vi "TB-Options Dialog.vi"(0 "Parameters in":T6={"Low cutoff (kHz)"=0.0, "High cutoff (kHz)"=0.0, "Duration (min)"=0.0, "dB SPL"=100.0, "Waveform"=enum."Noise", "WAVfile"=path "", "refWav"=path "", "use mic correction"=FALSE, "micCorrFile"=path "", "Pistonphone Level (dB SPL)"=0.0, "Sampling rate (Hz)"=0.0, "Buffer length (s)"=0.0, "Stream mic"=FALSE, "Fine adjust"={"Max"=0.0, "Min"=0.0}, "Mic gain"=0.0, "atten"=0.0, "Allow Slack"=FALSE, "max starts"=0, "Freq (kHz)"=8.0, "Tma (s)"=0.0, "Streamed"=[], "Drive"="", "Speaker"="", "Mic"="", "Analysis"={"Method"=enum."Default", "resol (Hz)"=0.0, "nfreq"=0, "signal"=""}, "exposeAtten"=0.0, "Digital"=""}, 2 "Parent VI":refnum<vi>) -> (4 "Parameters out":T6={"Low cutoff (kHz)"=0.0, "High cutoff (kHz)"=0.0, "Duration (min)"=0.0, "dB SPL"=100.0, "Waveform"=enum."Noise", "WAVfile"=path "", "refWav"=path "", "use mic correction"=FALSE, "micCorrFile"=path "", "Pistonphone Level (dB SPL)"=0.0, "Sampling rate (Hz)"=0.0, "Buffer length (s)"=0.0, "Stream mic"=FALSE, "Fine adjust"={"Max"=0.0, "Min"=0.0}, "Mic gain"=0.0, "atten"=0.0, "Allow Slack"=FALSE, "max starts"=0, "Freq (kHz)"=8.0, "Tma (s)"=0.0, "Streamed"=[], "Drive"="", "Speaker"="", "Mic"="", "Analysis"={"Method"=enum."Default", "resol (Hz)"=0.0, "nfreq"=0, "signal"=""}, "exposeAtten"=0.0, "Digital"=""}, 8 "Canceled?":bool)   [LabVIEW 2020]
uses:
  Typedefs/TB-Parameters.ctl
  Typedefs/TB-Analysis Parameters.ctl
  epl-vi-lib/Utility VIs/Buttons/KCheckmarkBoolean 2.ctl
  epl-vi-lib/Utility VIs/Controls/KBackground Gradient/KBackground Gradient.xctl
  epl-vi-lib/Utility VIs/Slack VIs/Slack/Slack.xctl
  epl-vi-lib/Utility VIs/Controls/KTable/KTable.xctl
  Typedefs/TB-User.ctl
  db6f5269-756f-40de-ad08-04ce0dc7adfb.vi
  epl-vi-lib/Utility VIs/File IO VIs/Read Write Anything/Read Anything.vi
panel:
  in  "Tab":T1(tab)
  in  "expose atten":dbl caption="Additional exposure attenuation (dB)"
  in  "max starts":i32 caption="Max number of starts (in case of error)"
  in  "Pistonphone Level":dbl caption="Pistonphone Level (dB SPL)"
  in  "Sampling rate (Hz)":dbl
  in  "Buffer length (s)":dbl
  in  "atten":dbl caption="Global attenuation (dB)"
  in  "Tma":dbl caption="Moving average (s)"
  in  "Signal":u16(ring)
  in  "Method":T2(ring)
  in  "resol":dbl caption="Spectrum resolution (Hz)"
  in  "nspect":i32 caption="Spectrum averages"
  in  "Digital":u16(ring) caption="Digital output" items=["None", "PXI1Slot3/port0/line0", "PXI1Slot3/port0/line1", "PXI1Slot3/port0/line2", "PXI1Slot3/port0/line3", "PXI1Slot3/port0/line4", "PXI1Slot3/port0/line5", "PXI1Slot3/port0/line6", "PXI1Slot3/port0/line7", "PXI1Slot4/port0/line0", "PXI1Slot4/port0/line1", "PXI1Slot4/port0/line2", "PXI1Slot4/port0/line3", "PXI1Slot4/port0/line4", "PXI1Slot4/port0/line5", "PXI1Slot4/port0/line6", "PXI1Slot4/port0/line7"]
  in  "Microphone":u16(ring) items=["PXI1Slot2/ai0", "PXI1Slot2/ai1", "PXI1Slot3/ai0", "PXI1Slot3/ai1", "PXI1Slot3/ai2", "PXI1Slot3/ai3", "PXI1Slot3/ai4", "PXI1Slot3/ai5", "PXI1Slot3/ai6", "PXI1Slot3/ai7", "PXI1Slot4/ai0", "PXI1Slot4/ai1", "PXI1Slot4/ai2", "PXI1Slot4/ai3", "PXI1Slot4/ai4", "PXI1Slot4/ai5", "PXI1Slot4/ai6", "PXI1Slot4/ai7"]
  in  "Speaker":u16(ring) items=["PXI1Slot2/ao0", "PXI1Slot2/ao1", "PXI1Slot3/ao0", "PXI1Slot3/ao1", "PXI1Slot4/ao0", "PXI1Slot4/ao1"]
  out "Cal mic":u16(xcontrol) caption="Additional signals"
  in  "Table":u16(xcontrol) caption="Additional signals"
  in  "Stream raw data to disk":T3
  in  "Add Button":bool
  in  "Users":i32(listbox)
  in  "Slack":cluster{"config":T4, "users":T5[]}(xcontrol)
  in  "Gradient":dbl(xcontrol)
  in  "Cancel":bool
  in  "OK":bool
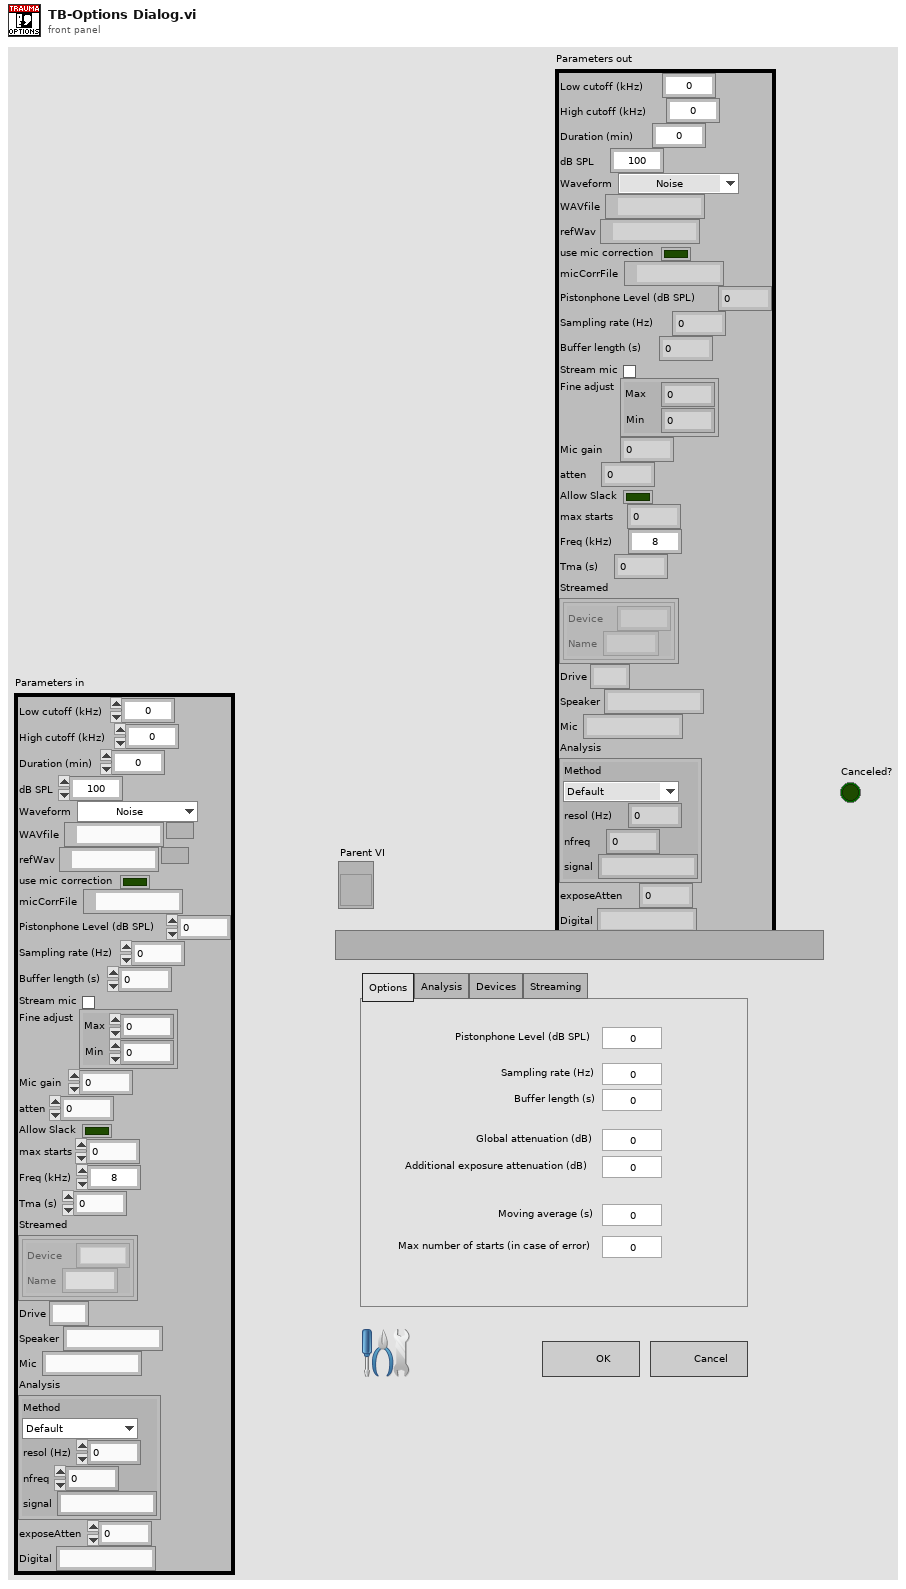
[diagram p1: front panel]
types:
  T1 = enum32{"Options", "Analysis", "Devices", "Streaming", "Slack"}
  T2 = enum16{"Default", "Periodogram", "Cross-spectrum"}
  T3 = typedef "KCheckmarkBoolean 2.ctl" = bool
  T4 = typedef "Slack-Configuration.ctl" = cluster{"app_id":string, "authed_user":cluster{"id":string}, "access_token":string, "bot_user_id":string, "team":cluster{"id":string, "name":string}, "bot channel":cluster{"id":string, "name":string}, "bot_user_name":string}
  T5 = typedef "Slack-User.ctl" = cluster{"id":string, "name":string}
  T6 = typedef "TB-Parameters.ctl" = cluster{"Low cutoff (kHz)":dbl, "High cutoff (kHz)":dbl, "Duration (min)":dbl, "dB SPL":dbl, "Waveform":enum16{"Noise", "File", "Tone"}, "WAVfile":path, "refWav":path, "use mic correction":bool, "micCorrFile":path, "Pistonphone Level (dB SPL)":dbl, "Sampling rate (Hz)":dbl, "Buffer length (s)":dbl, "Stream mic":bool, "Fine adjust":cluster{"Max":dbl, "Min":dbl}, "Mic gain":dbl, "atten":dbl, "Allow Slack":bool, "max starts":i32, "Freq (kHz)":dbl, "Tma (s)":dbl, "Streamed":cluster{"Device":string, "Name":string}[], "Drive":string, "Speaker":string, "Mic":string, "Analysis":T7, "exposeAtten":dbl, "Digital":string}
  T7 = typedef "TB-Analysis Parameters.ctl" = cluster{"Method":enum16{"Default", "Periodogram", "Cross-spectrum"}, "resol (Hz)":dbl, "nfreq":i32, "signal":string}
  T8 = enum8{"Enabled", "Disabled", "Disabled and Grayed Out"}
  T9 = typedef "TB-User.ctl" = cluster{"name":string, "id":string, "notify on errors":bool}
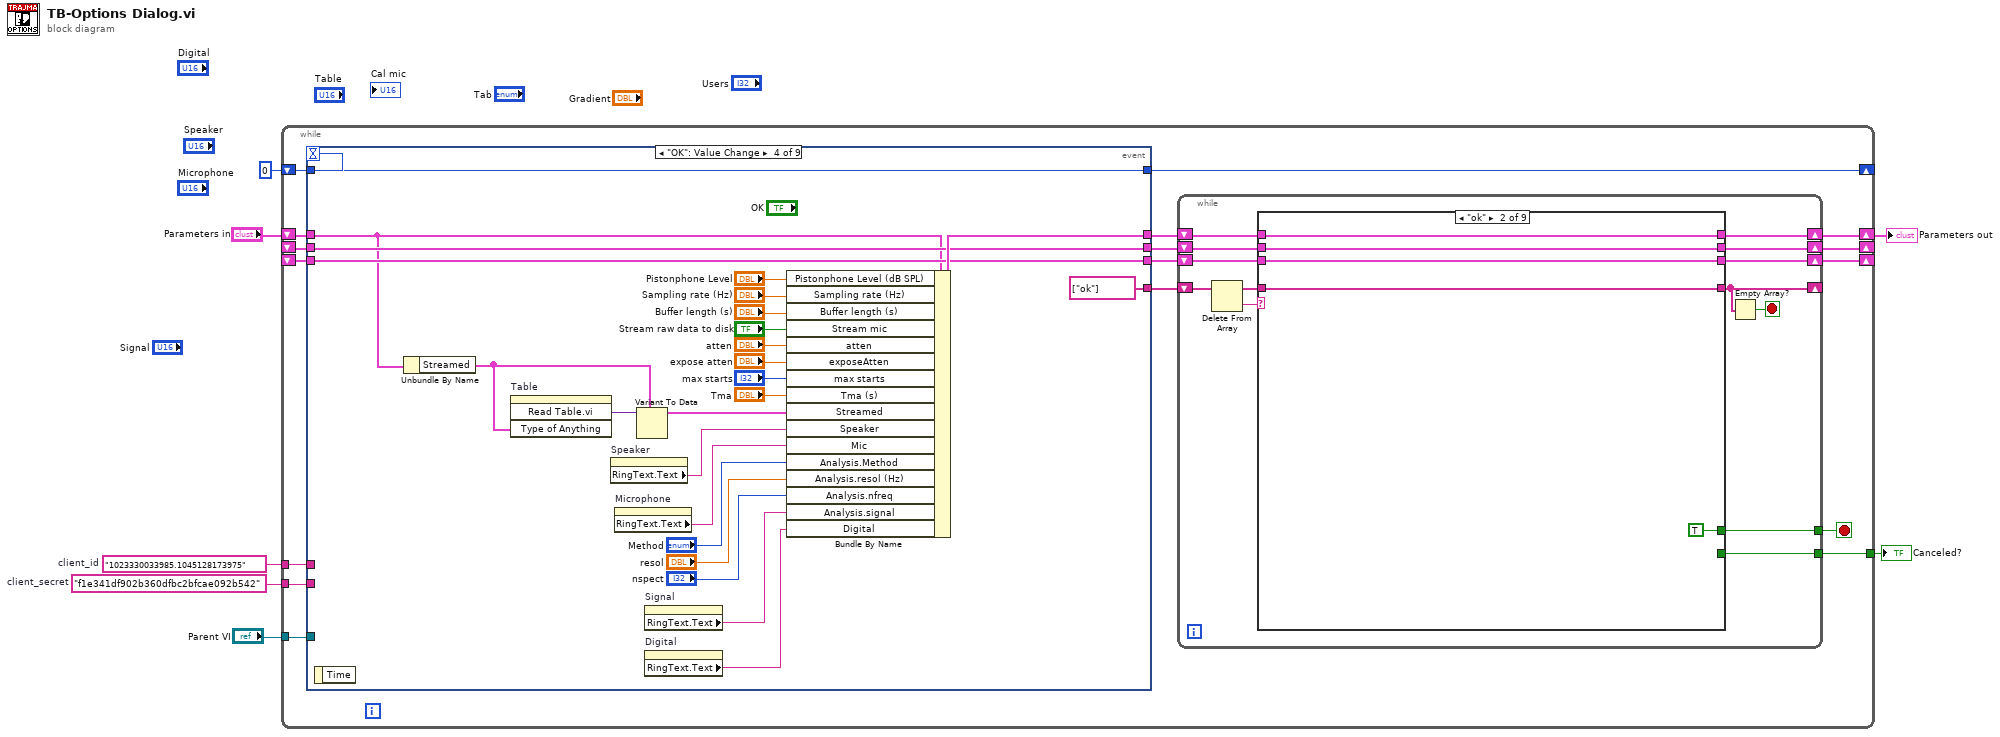
[diagram p0: block diagram]
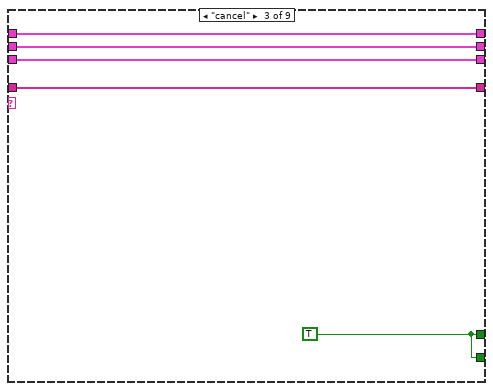
[diagram p3: hidden frame]
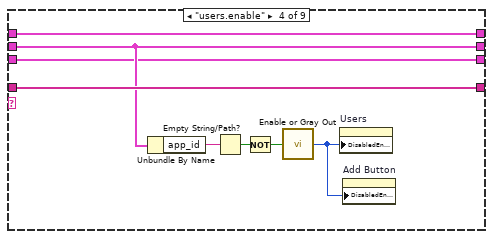
[diagram p4: hidden frame]
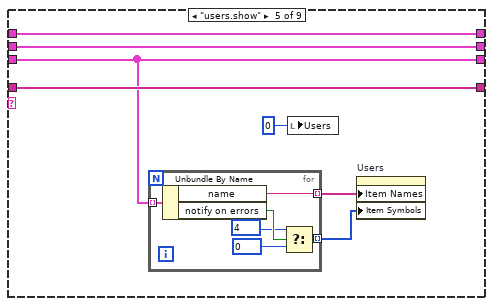
[diagram p5: hidden frame]
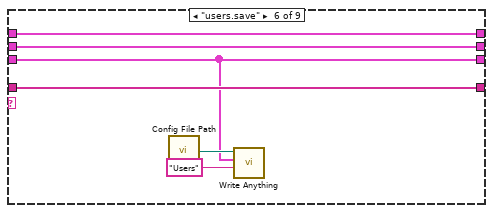
[diagram p6: hidden frame]
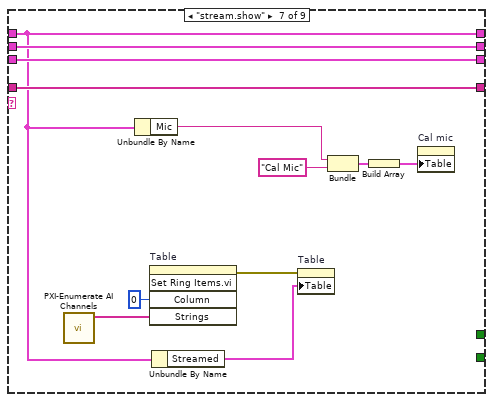
[diagram p7: hidden frame]
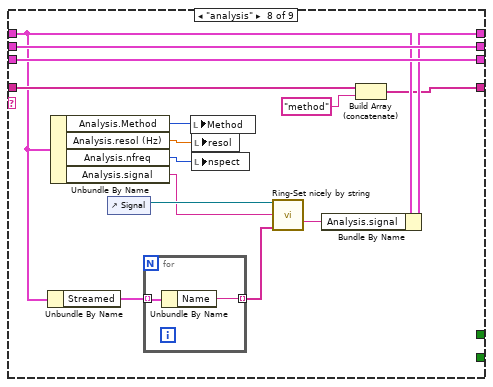
[diagram p8: hidden frame]
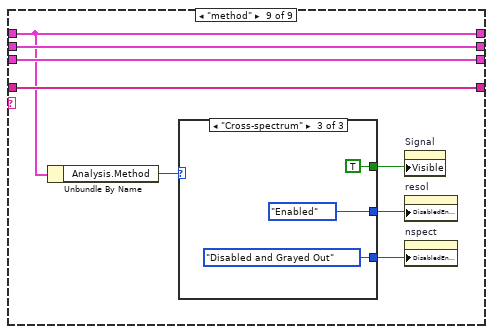
[diagram p9: hidden frame]
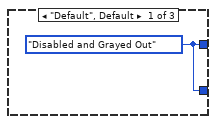
[diagram p10: hidden frame]
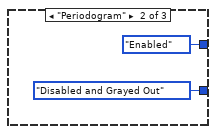
[diagram p11: hidden frame]
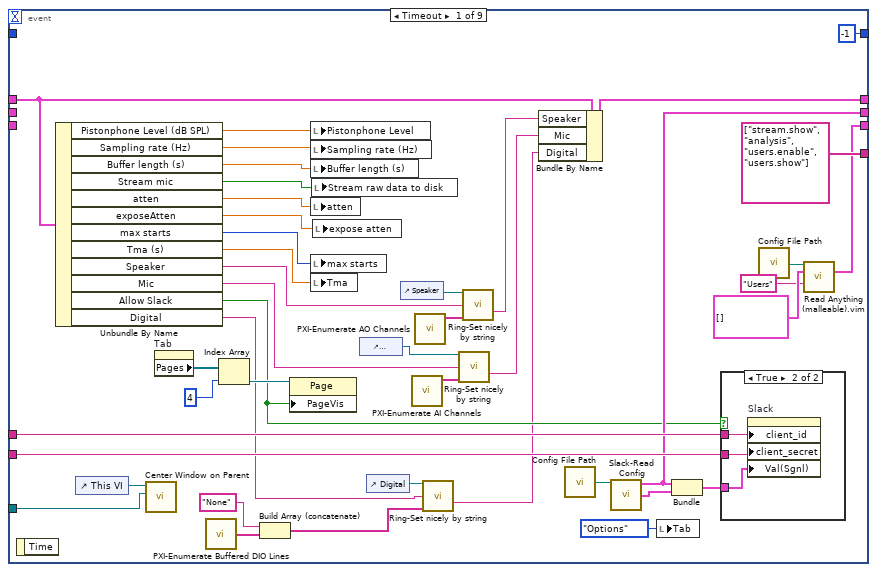
[diagram p12: hidden frame]
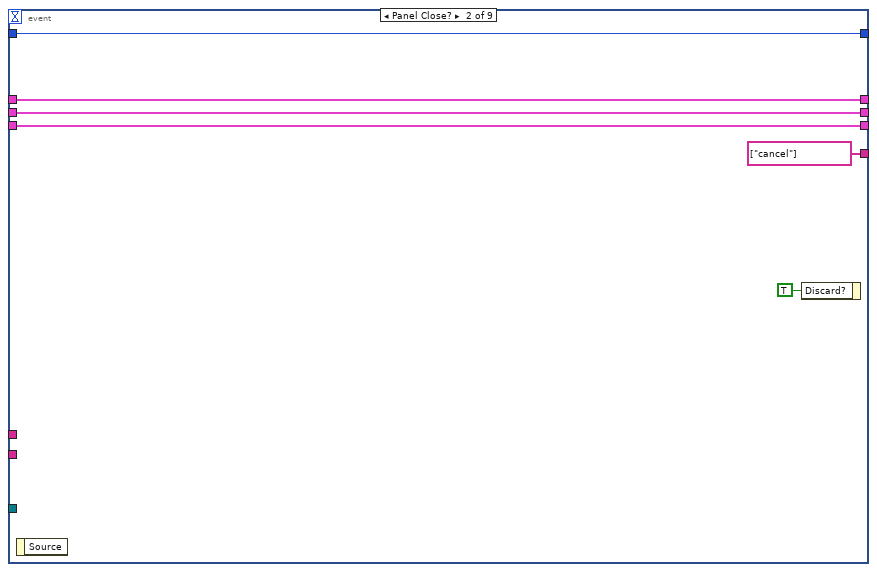
[diagram p14: hidden frame]
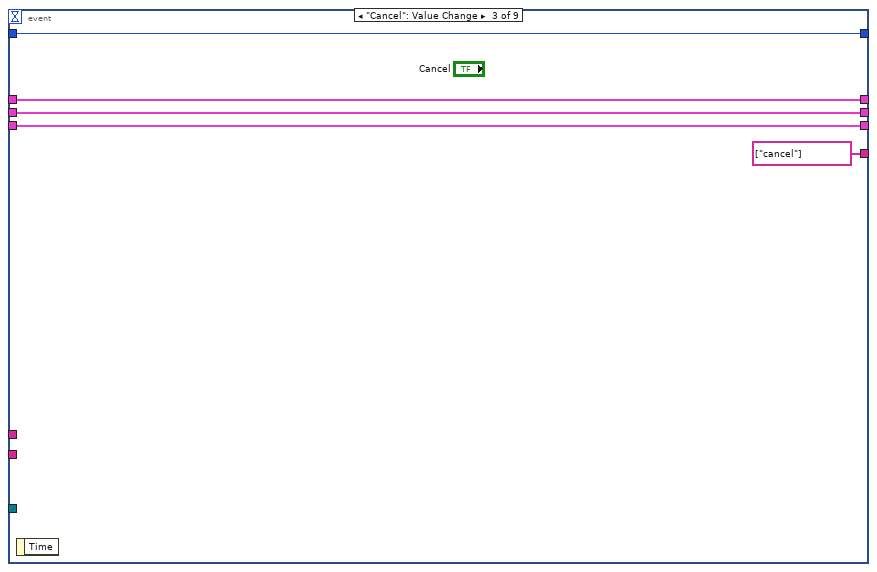
[diagram p15: hidden frame]
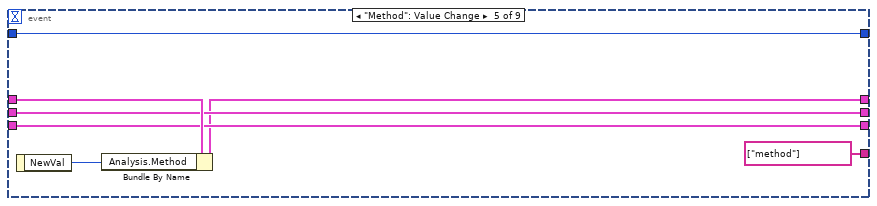
[diagram p16: hidden frame]
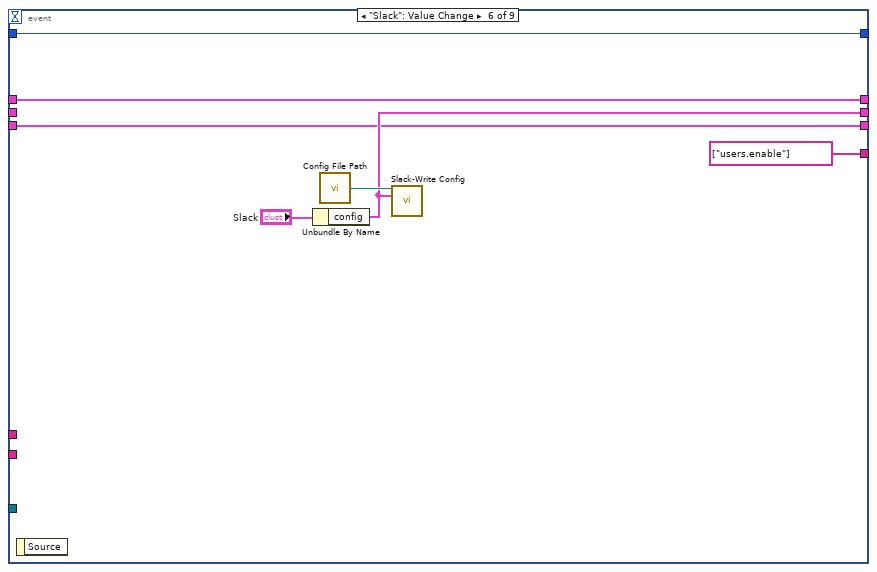
[diagram p17: hidden frame]
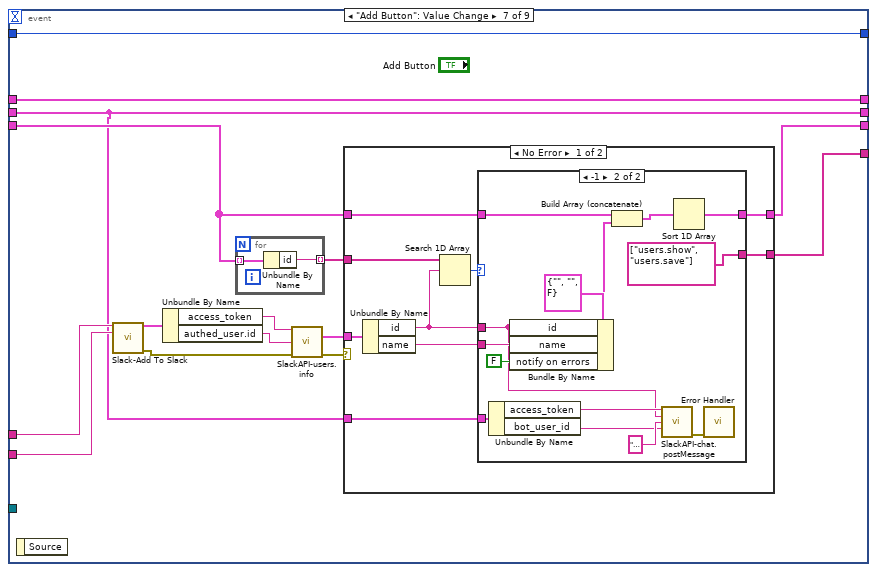
[diagram p18: hidden frame]
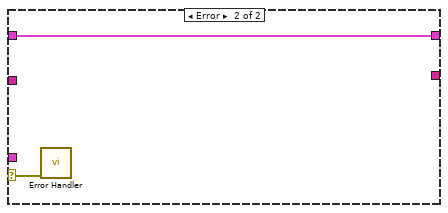
[diagram p20: hidden frame]
diagram:
  w1 = "f1e341df902b360dfbc2bfcae092b542"  # client_secret
  w2 = "1023330033985.1045128173975"  # client_id
  n1 = while {
    shift-right: [w24] -> _
    shift-left: 0 -> [w21]
    tunnel: [w11] -> w4
    shift-right: [w16] -> w5
    shift-left: "Parameters in" -> [w23]
    tunnel: "Parent VI" -> [w22]
    tunnel: w2 -> [w20]
    tunnel: w1 -> [w19]
    shift-right: [w14] -> _
    shift-left: _ -> [w13]
    shift-right: [w9] -> _
    shift-left: _ -> [w8]
    stop <- w12 stop-if-true
    n2 = event shown="[3] \"OK\": Value Change" {
      selector: _ -> [_ _ _ _ _ _ _ _ _]
      dyn-events: _ -> [_ _ _ _ _ _ _ _ _]
      timeout: w21 -> [_ _ _ _ _ _ _ _ _]
      tunnel: [-1 w173 w178 w196 w209 w215 w231 w268 w282] -> w24
      tunnel: w23 -> [w163 w172 w176 w190 w208 w216 w230 w267 w281]
      tunnel: [w136 w172 w176 w202 w204 w216 w230 w267 w281] -> w17
      tunnel: w22 -> [w156 _ _ _ _ _ _ _ _]
      tunnel: w21 -> [_ w173 w178 w196 w209 w215 w231 w268 w282]
      tunnel: w20 -> [w148 _ _ _ _ _ w225 _ _]
      tunnel: w19 -> [w147 _ _ _ _ _ w224 _ _]
      tunnel: [w146 w171 w175 w193 w207 w212 w217 w266 w275] -> w15
      tunnel: [string[] ["stream.show", "analysis", "users.enable", "users.show"] string[] ["cancel"] string[] ["cancel"] string[] ["ok"] string[] ["method"] string[] ["users.enable"] w218 _ w276] -> w18
      tunnel: w13 -> [_ w171 w175 w193 w207 _ w217 w266 w275]
      tunnel: [w129 w170 w174 w192 w206 w210 w219 w261 w277] -> w10
      tunnel: w8 -> [_ w170 w174 w192 w206 w210 w220 w261 w278]
      event Timeout {
        n3 = event-data() -> ()  [unwired: 1 in, 1 out]
        n4 = Unbundle By Name(w163) -> ("Pistonphone Level (dB SPL)"=w162:dbl, "Sampling rate (Hz)"=w161:dbl, "Buffer length (s)"=w160:dbl, "Stream mic"=w159:bool, "atten"=w158:dbl, "exposeAtten"=w128:dbl, "max starts"=w149:i32, "Tma (s)"=w144:dbl, "Speaker"=w140:string, "Mic"=w138:string, "Allow Slack"=w143:bool, "Digital"=w125:string)
        n5 = control-ref of="This VI"() -> (w157:refnum<vi>)
        n6 = call "Center Window on Parent.vi"("Parent VI"=w156, "VI in"=w157) -> ()  [unwired: 8 in, 2 out]
        n7 = property on="Tab" class="TabCtl (strict)"() -> ("Pages"=w155:refnum<vi>[])  [unwired: 2 in, 2 out]
        n8 = call "PXI-Enumerate Buffered DIO Lines.vi"() -> ("Buffered DIO"=w124:tag[])  [unwired: 14 in, 1 out]
        n9 = Index Array(array=w155, index=4) -> (element=w153:refnum<vi>)
        n10 = Build Array (concatenate)("None", w124) -> (w123:string[])
        n11 = property class="Page"(reference=w153, "PageVis"=w143) -> ()  [unwired: 1 in, 2 out]
        n12 = local write "Pistonphone Level"(w162) -> ()
        n13 = local write "Sampling rate (Hz)"(w161) -> ()
        n14 = local write "Buffer length (s)"(w160) -> ()
        n15 = local write "atten"(w158) -> ()
        n16 = local write "max starts"(w149) -> ()
        n17 = local write "Tma"(w144) -> ()
        n18 = local write "Stream raw data to disk"(w159) -> ()
        n19 = local write "expose atten"(w128) -> ()
        n20 = control-ref of="Microphone"() -> (w137:refnum<vi>)
        n21 = control-ref of="Digital"() -> (w127:refnum<vi>)
        n22 = control-ref of="Speaker"() -> (w142:refnum<vi>)
        n23 = call "PXI-Enumerate AI Channels.vi"() -> ("AI.PhysicalChans"=w139:tag[])  [unwired: 11 in]
        n24 = call "PXI-Enumerate AO Channels.vi"() -> ("AO.PhysicalChans"=w141:tag[])  [unwired: 11 in]
        n25 = call "Ring-Set nicely by string.vi"("Ring in"=w127, "Device"=w125, "Strings []"=w123) -> ("Selection"=w126:string)  [unwired: 8 in, 4 out]
        n26 = call "Ring-Set nicely by string.vi"("Ring in"=w137, "Device"=w138, "Strings []"=w139) -> ("Selection"=w134:string)  [unwired: 8 in, 4 out]
        n27 = call "Ring-Set nicely by string.vi"("Ring in"=w142, "Device"=w140, "Strings []"=w141) -> ("Selection"=w135:string)  [unwired: 8 in, 4 out]
        n28 = Bundle By Name(cluster=w163, "Speaker"=w135, "Mic"=w134, "Digital"=w126) -> (w136:T6)
        n29 = call "Config File Path.vi"() -> ("Default config file name"=w152:path)  [unwired: 1 in]
        n30 = call "Slack-Read Config.vi"("AppName"=w152) -> ("config"=w146:T4, "users"=w150:T5[])  [unwired: 12 in, 1 out]
        n31 = local write "Tab"(T1."Options" ("Tab")) -> ()
        n32 = Bundle("config"=w146, "users"=w150) -> (w151:cluster{"config":T4, "users":T5[]})  [unwired: 1 in]
        n33 = case shown="True" w143 {
          tunnel: w148 -> [_ w167]
          tunnel: w147 -> [_ w166]
          tunnel: w151 -> [_ w165]
          frame False {
          }
          frame True {
            n34 = property on="Slack" class="Slack (strict)"("client_id"=w167, "client_secret"=w166, "Val(Sgnl)"=w165) -> ()  [unwired: 2 in, 2 out]
          }
        }
        n35 = call "Config File Path.vi"() -> ("Default config file name"=w132:path)  [unwired: 1 in]
        n36 = call "Read Anything (malleable).vim"("Config file path"=w132, "Options in"=T9[] [] ("Array"), "Section"="Users" ("Section Name (Name of \"Anything\")")) -> ("Options out"=w129:T9[])  [unwired: 9 in, 3 out]
      }
      event Panel Close? {
        n37 = event-data() -> ()  [unwired: 1 in, 1 out]
        n38 = event-data("Discard?"=TRUE) -> ()  [unwired: 1 in, 1 out]
      }
      event "Cancel": Value Change {
        n39 = event-data() -> ()  [unwired: 1 in, 1 out]
      }
      event "OK": Value Change {
        n40 = event-data() -> ()  [unwired: 1 in, 1 out]
        n41 = Unbundle By Name(w190) -> ("Streamed"=w188:cluster{"Device":string, "Name":string}[])
        n42 = invoke on="Table" class="KTable (strict)" method="Read Table.vi"("Type of Anything"=w188) -> ("Read Table.vi"=w189:variant)  [unwired: 3 in, 3 out]
        n43 = property on="Speaker" class="Ring (strict)"() -> ("RingText.Text"=w186:string)  [unwired: 2 in, 2 out]
        n44 = property on="Microphone" class="Ring (strict)"() -> ("RingText.Text"=w185:string)  [unwired: 2 in, 2 out]
        n45 = Variant To Data(type=w188, Variant=w189) -> (data=w187:cluster{"Device":string, "Name":string}[])  [unwired: 1 in, 1 out]
        n46 = property on="Signal" class="Ring (strict)"() -> ("RingText.Text"=w181:string)  [unwired: 2 in, 2 out]
        n47 = property on="Digital" class="Ring (strict)"() -> ("RingText.Text"=w179:string)  [unwired: 2 in, 2 out]
        n48 = Bundle By Name(cluster=w190, "Pistonphone Level (dB SPL)"="Pistonphone Level", "Sampling rate (Hz)"="Sampling rate (Hz)", "Buffer length (s)"="Buffer length (s)", "Stream mic"="Stream raw data to disk", "atten"="atten", "exposeAtten"="expose atten", "max starts"="max starts", "Tma (s)"="Tma", "Streamed"=w187, "Speaker"=w186, "Mic"=w185, "Analysis.Method"="Method", "Analysis.resol (Hz)"="resol", "Analysis.nfreq"="nspect", "Analysis.signal"=w181, "Digital"=w179) -> (w202:T6)
      }
      event "Method": Value Change {
        n49 = event-data() -> ("NewVal"=w203:T2)  [unwired: 1 in]
        n50 = Bundle By Name(cluster=w208, "Analysis.Method"=w203) -> (w204:T6)
      }
      event "Slack": Value Change {
        n51 = event-data() -> ()  [unwired: 1 in, 1 out]
        n52 = Unbundle By Name("Slack") -> ("config"=w212:T4)
        n53 = call "Config File Path.vi"() -> ("Default config file name"=w213:path)  [unwired: 1 in]
        n54 = call "Slack-Write Config.vi"("AppName"=w213, "config"=w212) -> ()  [unwired: 13 in, 1 out]
      }
      event "Add Button": Value Change {
        n55 = event-data() -> ()  [unwired: 1 in, 1 out]
        n56 = call "Slack-Add To Slack.vi"("client_id"=w225, "client_secret"=w224) -> ("config"=w226:T4, "error out"=w228:errorcluster)  [unwired: 12 in]
        n57 = Unbundle By Name(w226) -> ("access_token"=w227:string, "authed_user.id"=w229:string)
        n58 = for {
          tunnel: w220 -> [w233] mode=indexing
          tunnel: [w232] -> w221 mode=indexing
          n59 = Unbundle By Name(w233) -> ("id"=w232:string)
        }
        n60 = call "SlackAPI-users.info.vi"("token"=w227, "user"=w229, "error in (no error)"=w228) -> ("user"=w222:T5, "error out"=w223:errorcluster)  [unwired: 10 in, 1 out]
        n61 = case shown="No Error" w223 {
          selector: w223 -> [_ w258]
          tunnel: w222 -> [w242 _]
          tunnel: w221 -> [w240 _]
          tunnel: w220 -> [w237 w259]
          tunnel: [w236 w259] -> w219
          tunnel: [w235 _] -> w218
          tunnel: w217 -> [w234 _]
          frame No Error {
            n62 = Unbundle By Name(w242) -> ("id"=w239:string, "name"=w241:string)
            n63 = Search 1D Array(1D array=w240, element=w239) -> (index of element=w238:i32)  [unwired: 1 in]
            n64 = case shown="-1" w238 {
              tunnel: w241 -> [_ w256]
              tunnel: w239 -> [_ w245]
              tunnel: w237 -> [w243 w254]
              tunnel: [w243 w250] -> w236
              tunnel: [_ string[] ["users.show", "users.save"]] -> w235
              tunnel: w234 -> [_ w249]
              frame 0, Default {
              }
              frame -1 {
                n65 = Unbundle By Name(w249) -> ("access_token"=w248:string, "bot_user_id"=w246:string)
                n66 = Bundle By Name(cluster=T9 {"name"="", "id"="", "notify on errors"=FALSE} ("User"), "id"=w245, "name"=w256, "notify on errors"=FALSE ("always notify")) -> (w253:T9)
                n67 = Build Array (concatenate)(w254, w253) -> (w251:T9[])
                n68 = call "SlackAPI-chat.postMessage.vi"("access_token"=w248, "user ID"=w245, "message"="You've been added to the Trauma Box users.", "username"=w246) -> ("error out"=w244:errorcluster)  [unwired: 11 in]
                n69 = Sort 1D Array(array=w251) -> (sorted array=w250:T9[])
                n70 = call "Error Handler.vi"("error in (no error)"=w244) -> ()  [unwired: 12 in, 3 out]
              }
            }
          }
          frame Error {
            n71 = call "Error Handler.vi"("error in (no error)"=w258) -> ()  [unwired: 12 in, 3 out]
          }
        }
      }
      event "Users": Shortcut Menu Activation? {
        n72 = event-data() -> ("MenuRef"=w263:refnum<k9>)  [unwired: 1 in]
        n73 = local read "Users"() -> (w262:i32)
        n74 = Less Than 0?(x=w262) -> (x < 0?=w264:bool)
        n75 = Empty Array?(array=w261) -> (empty?=w265:bool)
        n76 = Or(x=w265, y=w264) -> (x .or. y?=w260:bool)
        n77 = case shown="False" w260 {
          tunnel: w263 -> [w271 _]
          tunnel: w262 -> [w273 _]
          tunnel: w261 -> [w274 _]
          frame False {
            n78 = Index Array(array=w274, index=w273) -> (element=w272:T9)
            n79 = Unbundle By Name(w272) -> ("notify on errors"=w269:bool)
            n80 = Set Menu Item Info(6:w269, 7:"cmAlwaysNotify" ("item tag"), 11:w271) -> ()  [unwired: 4 in, 2 out]
          }
          frame True {
          }
        }
        n81 = event-data("Discard?"=w260) -> ()  [unwired: 1 in, 1 out]
      }
      event "Users": Shortcut Menu Selection (User) {
        n82 = event-data() -> ("ItemTag"=w280:string)  [unwired: 1 in]
        n83 = local read "Users"() -> (w279:i32)
        n84 = case shown="\"cmRemoveUser\"" w280 {
          tunnel: w278 -> [w283 w288 w303]
          tunnel: w279 -> [_ w286 w302]
          tunnel: [w283 w285 w300] -> w277
          tunnel: [_ string[] ["users.show", "users.save"] string[] ["users.show", "users.save"]] -> w276
          tunnel: w275 -> [_ _ w295]
          frame "", Default {
          }
          frame "cmAlwaysNotify" {
            n85 = Index Array(array=w288, index=w286) -> (element=w290:T9)
            n86 = Unbundle By Name(w290) -> ("notify on errors"=w291:bool)
            n87 = Not(x=w291) -> (.not. x?=w289:bool)
            n88 = Bundle By Name(cluster=w290, "notify on errors"=w289) -> (w287:T9)
            n89 = Replace Array Subset(array=w288, new element=w287, index=w286) -> (w285:T9[])
          }
          frame "cmRemoveUser" {
            n90 = Delete From Array(array=w303, length=1, index=w302) -> (deleted portion=w294:T9[], array with subset deleted=w300:T9[])
            n91 = Index Array(array=w294) -> (element=w293:T9)  [unwired: 1 in]
            n92 = Unbundle By Name(w295) -> ("access_token"=w299:string, "bot_user_id"=w297:string)
            n93 = Unbundle By Name(w293) -> ("id"=w292:string)
            n94 = call "SlackAPI-chat.postMessage.vi"("access_token"=w299, "user ID"=w292, "message"="You've been removed from the Trauma Box users.", "username"=w297) -> ("error out"=w296:errorcluster)  [unwired: 11 in]
            n95 = call "Error Handler.vi"("error in (no error)"=w296) -> ()  [unwired: 12 in, 3 out]
          }
        }
      }
    }
    n96 = while {
      shift-right: [w34] -> _
      shift-left: w18 -> [w37]
      shift-right: [w31] -> w16
      shift-left: w17 -> [w32]
      shift-right: [w29] -> w14
      shift-left: w15 -> [w30]
      tunnel: [w28] -> w12
      tunnel: [w27] -> w11
      shift-right: [w25] -> w9
      shift-left: w10 -> [w26]
      stop <- w33 stop-if-true
      n97 = Delete From Array(array=w37) -> (deleted portion=w35:string, array with subset deleted=w36:string[])  [unwired: 2 in]
      n98 = case shown="\"ok\"" w35 {
        tunnel: w36 -> [w41 w46 w51 w59 w66 w78 w90 w105 w115]
        tunnel: [w41 w46 w51 w59 w66 w78 w90 w92 w115] -> w34
        tunnel: w32 -> [w40 w45 w50 w58 w65 w77 w80 w101 w112]
        tunnel: [w40 w45 w50 w58 w65 w77 w80 w97 w112] -> w31
        tunnel: w30 -> [w39 w44 w49 w57 w64 w76 w89 w104 w114]
        tunnel: [w39 w44 w49 w57 w64 w76 w89 w104 w114] -> w29
        tunnel: [_ TRUE w48 _ _ _ _ _ _] -> w28
        tunnel: [_ _ w48 _ _ _ _ _ _] -> w27
        tunnel: w26 -> [w38 w42 w47 w52 w63 w74 w88 w103 w113]
        tunnel: [w38 w42 w47 w52 w63 w74 w88 w103 w113] -> w25
        frame "", Default {
        }
        frame "ok" {
        }
        frame "cancel" {
          w48 = TRUE
        }
        frame "users.enable" {
          n99 = Unbundle By Name(w57) -> ("app_id"=w56:string)
          n100 = Empty String/Path?(string/path=w56) -> (empty?=w55:bool)
          n101 = Not(x=w55) -> (.not. x?=w54:bool)
          n102 = call "Enable or Gray Out.vi"("Boolean"=w54) -> ("Disabled"=w53:T8)
          n103 = property on="Users" class="LstBox (strict)"("DisabledEnum"=w53) -> ()  [unwired: 2 in, 2 out]
          n104 = property on="Add Button" class="Bool"("DisabledEnum"=w53) -> ()  [unwired: 2 in, 2 out]
        }
        frame "users.show" {
          n105 = for {
            tunnel: w63 -> [w72] mode=indexing
            tunnel: [w71] -> w62 mode=indexing
            tunnel: [w68] -> w60 mode=indexing
            n106 = Unbundle By Name(w72) -> ("name"=w71:string, "notify on errors"=w70:bool)
            n107 = Select(t=4, s=w70, f=0) -> (s? t:f=w68:i32)
          }
          n108 = local write "Users"(0) -> ()
          n109 = property on="Users" class="LstBox (strict)"("Item Names"=w62, "Item Symbols"=w60) -> ()  [unwired: 2 in, 2 out]
        }
        frame "users.save" {
          n110 = call "Config File Path.vi"() -> ("Default config file name"=w75:path)  [unwired: 1 in]
          n111 = call "Write Anything.vi"("Section Name (Name of \"Anything\")"="Users" ("Section Name (Name of \"Anything\")"), "Anything"=w74, "Path (dialog)"=w75) -> ()  [unwired: 7 in, 2 out]
        }
        frame "stream.show" {
          n112 = call "PXI-Enumerate AI Channels.vi"() -> ("AI.PhysicalChans"=w83:tag[])  [unwired: 11 in]
          n113 = Unbundle By Name(w80) -> ("Mic"=w79:string)
          n114 = invoke on="Table" class="KTable (strict)" method="Set Ring Items.vi"("Column"=0, "Strings"=w83) -> (error out=w82:errorcluster)  [unwired: 3 in, 4 out]
          n115 = Unbundle By Name(w80) -> ("Streamed"=w81:cluster{"Device":string, "Name":string}[])
          n116 = property on="Table" class="KTable (strict)"(error in=w82, "Table"=w81) -> ()  [unwired: 1 in, 2 out]
          n117 = Bundle("Mic"=w79, "Cal Mic") -> (w85:cluster{"Mic":string, string})  [unwired: 1 in]
          n118 = Build Array(w85) -> (w84:cluster{"Mic":string, string}[])
          n119 = property on="Cal mic" class="KTable (strict)"("Table"=w84) -> ()  [unwired: 2 in, 2 out]
        }
        frame "analysis" {
          n120 = Unbundle By Name(w101) -> ("Streamed"=w102:cluster{"Device":string, "Name":string}[])
          n121 = Unbundle By Name(w101) -> ("Analysis.Method"=w100:T2, "Analysis.resol (Hz)"=w99:dbl, "Analysis.nfreq"=w98:i32, "Analysis.signal"=w94:string)
          n122 = control-ref of="Signal"() -> (w96:refnum<vi>)
          n123 = for {
            tunnel: w102 -> [w107] mode=indexing
            tunnel: [w106] -> w95 mode=indexing
            n124 = Unbundle By Name(w107) -> ("Name"=w106:string)
          }
          n125 = local write "Method"(w100) -> ()
          n126 = local write "resol"(w99) -> ()
          n127 = local write "nspect"(w98) -> ()
          n128 = call "Ring-Set nicely by string.vi"("Ring in"=w96, "Device"=w94, "Strings []"=w95) -> ("Selection"=w93:string)  [unwired: 8 in, 4 out]
          n129 = Bundle By Name(cluster=w101, "Analysis.signal"=w93) -> (w97:T6)
          n130 = Build Array (concatenate)(w105, "method") -> (w92:string[])
        }
        frame "method" {
          n131 = Unbundle By Name(w112) -> ("Analysis.Method"=w111:T2)
          n132 = case shown="\"Cross-spectrum\"" w111 {
            tunnel: [_ _ TRUE] -> w110
            tunnel: [w116 T8."Enabled" ("Disabled") T8."Enabled" ("Disabled")] -> w109
            tunnel: [w116 T8."Disabled and Grayed Out" ("Disabled") T8."Disabled and Grayed Out" ("Disabled")] -> w108
            frame "Default", Default {
              w116 = T8."Disabled and Grayed Out" ("Disabled")
            }
            frame "Periodogram" {
            }
            frame "Cross-spectrum" {
            }
          }
          n133 = property on="Signal" class="Ring (strict)"("Visible"=w110) -> ()  [unwired: 2 in, 2 out]
          n134 = property on="resol" class="DigNum (strict)"("DisabledEnum"=w109) -> ()  [unwired: 2 in, 2 out]
          n135 = property on="nspect" class="DigNum (strict)"("DisabledEnum"=w108) -> ()  [unwired: 2 in, 2 out]
        }
      }
      n136 = Empty Array?(array=w34) -> (empty?=w33:bool)
    }
  }
  "Parameters out" <- w5
  "Canceled?" <- w4
